vi "SelectionListToOrder.vi"(9 "AnalysisResultNum":i32=3, 11 "SelectionList":T1[](array[typedef])) -> (3 "Order":i32[](array[numeric]))   [LabVIEW 2019]
uses:
  Controls/SelectionListEntry.ctl
  Controls/SelectionListEntryPointType.ctl
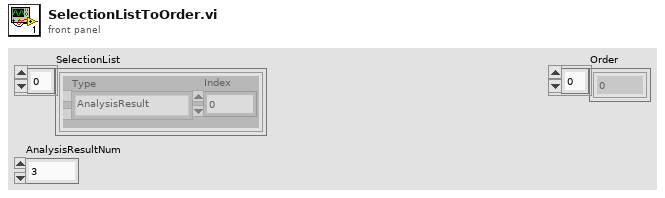
[diagram p1: front panel]
types:
  T1 = typedef "SelectionListEntry.ctl" = cluster{"Type":T2, "Index":i32}
  T2 = typedef "SelectionListEntryPointType.ctl" = enum16{"AnalysisResult", "CaliperResult"}
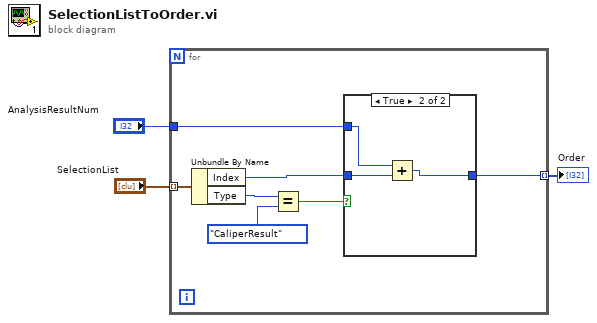
[diagram p0: block diagram]
diagram:
  n1 = for {
    tunnel: "SelectionList" -> [w10] mode=indexing
    tunnel: "AnalysisResultNum" -> [w6]
    tunnel: [w4] -> w1 mode=indexing
    n2 = Unbundle By Name(w10) -> ("Index"=w5:i32, "Type"=w9:T2)
    n3 = Equal?(x=w9, y=SelectionListEntryPointType."CaliperResult" ("Type")) -> (x = y?=w7:bool)
    n4 = case shown="True" w7 {
      tunnel: w6 -> [_ w14]
      tunnel: w5 -> [w11 w13]
      tunnel: [w11 w12] -> w4
      frame False {
      }
      frame True {
        n5 = Add(x=w14, y=w13) -> (x+y=w12:i32)
      }
    }
  }
  "Order" <- w1
